vi "PathPlanner_PathFinder_WorkerThreadALT.vi"() -> ()   [LabVIEW 2019, in "PathPlanner24.lvlib"]
doc: "Background worker VI (thread) for the Path Finder / Path Finding functions. This will be started by the New function. This should NOT be called by an end user."
uses:
  PathPlanner24.lvlib
  PathPlanner_GridPosition_Get.vi
  <vilib>/Utility/error.llb/Clear Errors.vi
  PathPlanner_PathFinder_SetNewPathAvail.vi
  PathPlanner_PathFinder_ExtractPath.vi
  PathPlanner_GridPosition_Equals.vi
  PathPlanner_PathFinder_GridPosToTranslation2d.vi
  PathPlanner_PathFinder_ApplyControlSmooth.vi
  PathPlanner_PathFinder_ExtractPathSub1ALT.vi
  PathPlanner_PathFinder_IsWalkable.vi
  PathPlanner_PathFinder_ApplyAnchorSmooth.vi
  <vilib>/Rock Robotics/WPI/ThirdParty/JAS_Junk/TrajLib/Translation2d_GetDistance.vi
  PathPlanner_PathFinder_Constants.vi
  <vilib>/Rock Robotics/WPI/ThirdParty/JAS_Junk/TrajLib/Translation2d_Create_DistAng.vi
  <vilib>/Rock Robotics/WPI/ThirdParty/JAS_Junk/TrajLib/Translation2d_Minus.vi
  <vilib>/Rock Robotics/WPI/ThirdParty/JAS_Junk/TrajLib/Translation2d_GetAngle.vi
  <vilib>/Rock Robotics/WPI/ThirdParty/JAS_Junk/TrajLib/Translation2d_Plus.vi
  <vilib>/Rock Robotics/WPI/ThirdParty/JAS_Junk/TrajLib/Translation2d_Create.vi
  <vilib>/Rock Robotics/WPI/ThirdParty/JAS_Junk/TrajLib/Translation2d_Times.vi
  PathPlanner_GridPosition_New.vi
  <vilib>/Rock Robotics/WPI/ThirdParty/JAS_Junk/TrajLib/Util_CalcDist.vi
  <vilib>/Rock Robotics/WPI/ThirdParty/JAS_Junk/TrajLib/Rotation2d_GetAngleCosSin.vi
  <vilib>/Rock Robotics/WPI/ThirdParty/JAS_Junk/TrajLib/Translation2d_GetXY.vi
  <vilib>/Rock Robotics/WPI/ThirdParty/JAS_Junk/TrajLib/Rotation2d_CreateXY.vi
  <vilib>/robotics/Navigation/shared/MapNode/OccupancyGridNode/NI_Robotics_OccupancyGridMapNode.lvclass
  C:/Program Files/National Instruments/LabVIEW 2019/vi.lib/robotics/Navigation/shared/MapNode/AbstractDstarNode/NI_Robotics_AbstractDstarNode.lvclass
  <vilib>/robotics/Navigation/shared/WorldMap/OccupancyGridWorldMap/NI_Robotics_OccupancyGridWorldMap.lvclass
  C:/Program Files/National Instruments/LabVIEW 2019/vi.lib/robotics/Navigation/shared/WorldMap/AbstractDstarWorldMap/NI_Robotics_AbstractDstarWorldMap.lvclass
  <vilib>/robotics/Navigation/shared/MapNode/AbstractDstarNode/NI_Robotics_AbstractDstarNode.lvclass
  C:/Program Files/National Instruments/LabVIEW 2019/vi.lib/robotics/Navigation/shared/MapNode/AbstractAstarNode/NI_Robotics_AbstractAstarNode.lvclass
  PathPlanner_PathFinder_Globals.vi
  <vilib>/robotics/Navigation/shared/WorldMap/OccupancyGridWorldMap/Get Cell Reference.vi
  <vilib>/robotics/Navigation/Anytime D Star/Anytime D Star Initialize.vi
  <vilib>/robotics/Navigation/Anytime D Star/Anytime D Star Plan.vi
  <vilib>/robotics/Navigation/shared/WorldMap/OccupancyGridWorldMap/Get Cells in Path.vi
panel:
  in  "Main Name":string
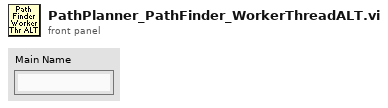
[diagram p1: front panel]
types:
  T1 = typedef "Semaphore RefNum" = refnum<k1>
  T2 = enum32{"Bad", "Idle", "Run top level", "Running"}
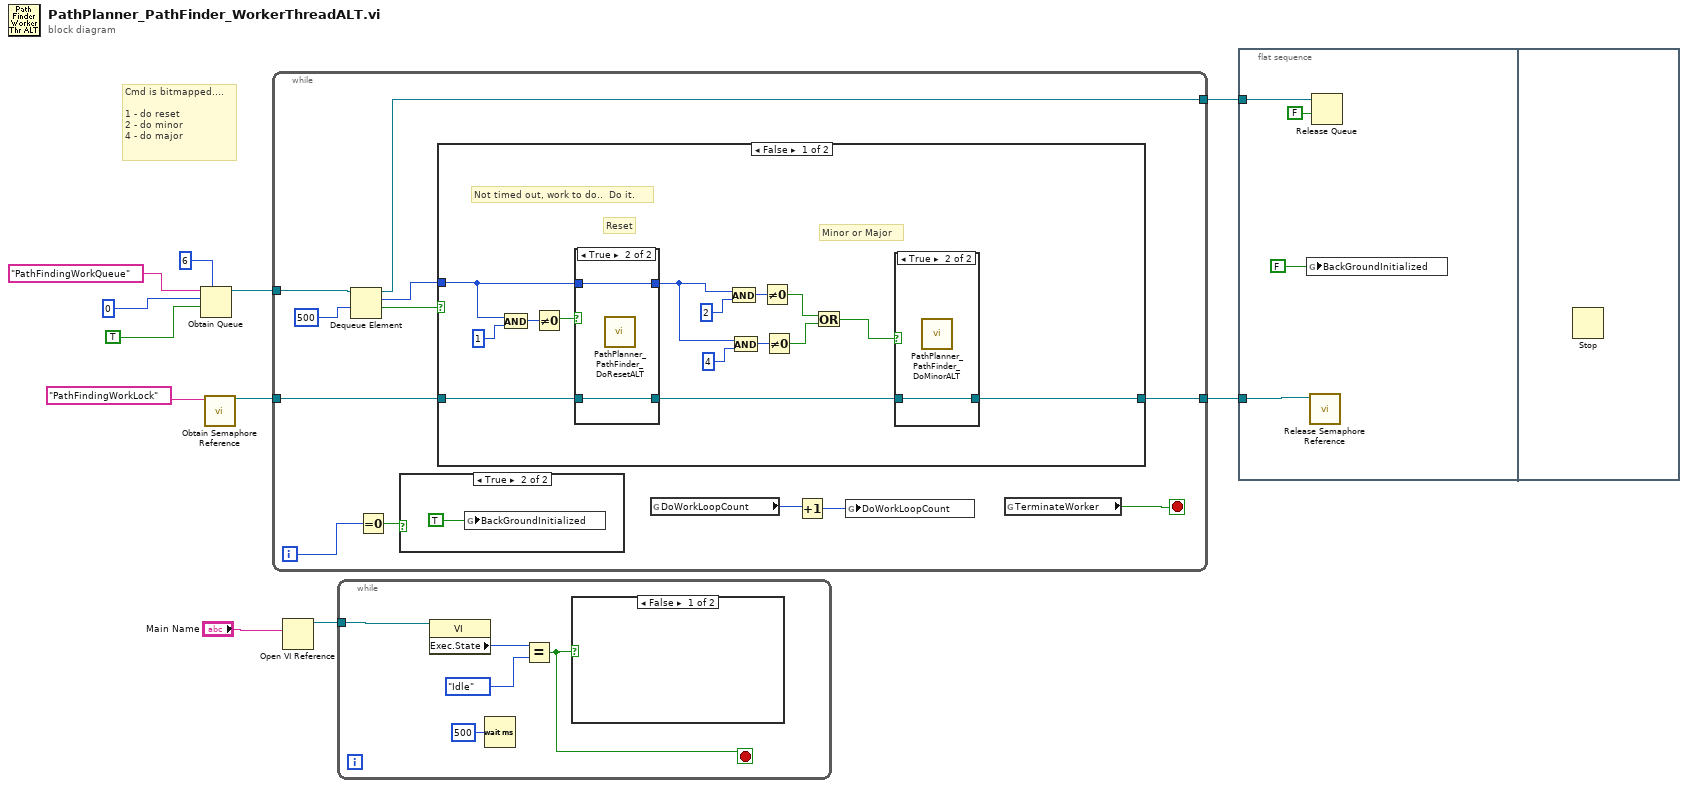
[diagram p0: block diagram]
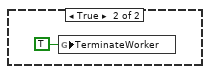
[diagram p2: hidden frame]
diagram:
  # "Cmd is bitmapped....\n\n1 - do reset\n2 - do minor\n4 - do major"
  n1 = Obtain Queue(max queue size (-1, unlimited)=6, name (unnamed)="PathFindingWorkQueue", element data type=0, create if not found? (T)=TRUE) -> (queue out=w3:refnum<queue>)  [unwired: 1 in, 2 out]
  n2 = call <vilib>:"Obtain Semaphore Reference.vi"("name (unnamed)"="PathFindingWorkLock") -> ("semaphore"=w5:T1)  [unwired: 4 in, 2 out]
  n3 = while {
    tunnel: w3 -> [w22]
    tunnel: [w18] -> w7
    tunnel: w5 -> [w17]
    tunnel: [w16] -> w4
    i -> [w13]
    stop <- w23 stop-if-true
    n4 = Dequeue Element(queue=w22, timeout in ms (-1)=500) -> (queue out=w18:refnum<queue>, element=w19:i32, timed out?=w20:bool)  [unwired: 1 in, 1 out]
    n5 = Equal To 0?(x=w13) -> (x = 0?=w12:bool)
    n6 = case shown="True" w12 {
      frame False {
      }
      frame True {
        n7 = global write "PathPlanner_PathFinder_Globals.vi" "BackGroundInitialized"(TRUE ("TerminateWorker")) -> ()
      }
    }
    n8 = case shown="False" w20 {
      tunnel: w19 -> [w34 _]
      tunnel: w17 -> [w31 w46]
      tunnel: [w29 w46] -> w16
      frame False {
        # "Minor or Major"
        # "Reset"
        # "Not timed out, work to do..  Do it."
        n9 = And(x=w34, y=1) -> (x .and. y?=w37:i32)
        n10 = Not Equal To 0?(x=w37) -> (x != 0?=w38:bool)
        n11 = case shown="True" w38 {
          tunnel: w34 -> [w43 w45]
          tunnel: [w43 w45] -> w28
          tunnel: w31 -> [w42 w44]
          tunnel: [w42 w44] -> w30
          frame False {
          }
          frame True {
            n12 = call "PathPlanner_PathFinder_DoResetALT.vi"() -> ()  [unwired: 11 in, 1 out]
          }
        }
        n13 = And(x=w28, y=2) -> (x .and. y?=w35:i32)
        n14 = And(x=w28, y=4) -> (x .and. y?=w32:i32)
        n15 = Not Equal To 0?(x=w35) -> (x != 0?=w27:bool)
        n16 = Not Equal To 0?(x=w32) -> (x != 0?=w26:bool)
        n17 = Or(x=w27, y=w26) -> (x .or. y?=w25:bool)
        n18 = case shown="True" w25 {
          tunnel: w30 -> [w40 w41]
          tunnel: [w40 w41] -> w29
          frame False {
          }
          frame True {
            n19 = call "PathPlanner_PathFinder_DoMinorALT.vi"() -> ()  [unwired: 11 in, 1 out]
          }
        }
      }
      frame True {
        # "#TODO  Add I'm alive counter"
        # "Timed out, no work to do...."
      }
    }
    n20 = global read "PathPlanner_PathFinder_Globals.vi" "DoWorkLoopCount"() -> (w15:i64)
    n21 = Increment(x=w15) -> (x+1=w14:i64)
    n22 = global write "PathPlanner_PathFinder_Globals.vi" "DoWorkLoopCount"(w14) -> ()
    n23 = global read "PathPlanner_PathFinder_Globals.vi" "TerminateWorker"() -> (w23:bool)
  }
  n24 = Open VI Reference(vi path="Main Name") -> (vi reference=w1:refnum<vi>)  [unwired: 5 in, 1 out]
  n25 = while {
    tunnel: w1 -> [w48]
    stop <- w49 stop-if-true
    n26 = property class="VI"(reference=w48) -> ("Exec.State"=w51:T2)  [unwired: 1 in, 2 out]
    n27 = Wait (ms)(milliseconds to wait=u32 500) -> ()  [unwired: 1 out]
    n28 = Equal?(x=w51, y=T2."Idle") -> (x = y?=w49:bool)
    n29 = case shown="False" w49 {
      frame False {
      }
      frame True {
        n30 = global write "PathPlanner_PathFinder_Globals.vi" "TerminateWorker"(TRUE ("TerminateWorker")) -> ()
      }
    }
  }
  n31 = flat-sequence {
    tunnel: w7 -> [w56]
    tunnel: w4 -> [w54]
    frame #0 {
      n32 = global write "PathPlanner_PathFinder_Globals.vi" "BackGroundInitialized"(FALSE ("TerminateWorker")) -> ()
      n33 = call <vilib>:"Release Semaphore Reference.vi"("semaphore"=w54) -> ()  [unwired: 9 in, 2 out]
      n34 = Release Queue(queue=w56, force destroy? (F)=FALSE) -> ()  [unwired: 1 in, 3 out]
    }
    frame #1 {
      n35 = Stop() -> ()  [unwired: 1 in]
    }
  }
